vi "PI Update PF Indicator.vi"(6 "PFLabel":refnum<vi>, 7 "Warn Text":string, 8 "Warn? (f)":bool, 9 "Pass? (f)":bool, 11 "error in (no error)":errorcluster) -> (1 "Status Text":string, 3 "error out":errorcluster)   [LabVIEW 2011]
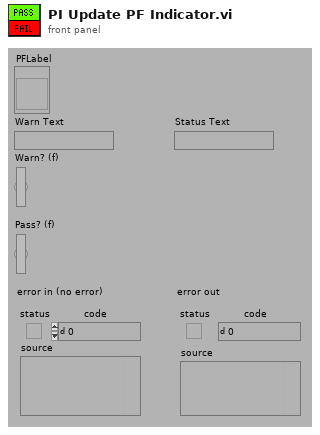
[diagram p1: front panel]
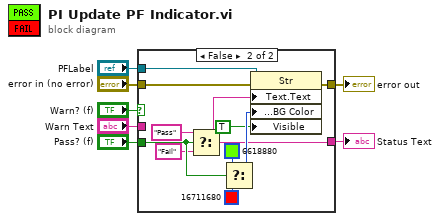
[diagram p0: block diagram]
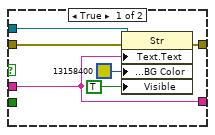
[diagram p2: hidden frame]
diagram:
  n1 = case shown="False" "Warn? (f)" {
    tunnel: "error in (no error)" -> [w13 w24]
    tunnel: "PFLabel" -> [w12 w23]
    tunnel: [w10 w18] -> w5
    tunnel: "Pass? (f)" -> [_ w17]
    tunnel: [w8 w16] -> w2
    tunnel: "Warn Text" -> [w8 _]
    frame True {
      n2 = property class="Str"(reference=w12, error in=w13, "Text.Text"=w8, "Text.Text Colors:BG Color"=u32 13158400, "Visible"=TRUE) -> (error out=w10:errorcluster)  [unwired: 1 out]
    }
    frame False {
      n3 = Select(t="Pass", s=w17, f="Fail") -> (s? t:f=w16:string)
      n4 = Select(t=u32 6618880, s=w17, f=u32 16711680) -> (s? t:f=w20:u32)
      n5 = property class="Str"(reference=w23, error in=w24, "Text.Text"=w16, "Text.Text Colors:BG Color"=w20, "Visible"=TRUE) -> (error out=w18:errorcluster)  [unwired: 1 out]
    }
  }
  "error out" <- w5
  "Status Text" <- w2
